vi "galvo_set_channels.vi"(8 "error in (no error)":errorcluster, 9 "y_channel":tag, 10 "x_channel":tag, 11 "galvo in":refnum<class "galvo.lvclass">) -> (0 "error out":errorcluster, 3 "galvo out":refnum<class "galvo.lvclass">)   [LabVIEW 2015, in "galvo.lvclass"]
uses:
  galvo.lvclass
  galvo.lvclass/galvo.ctl
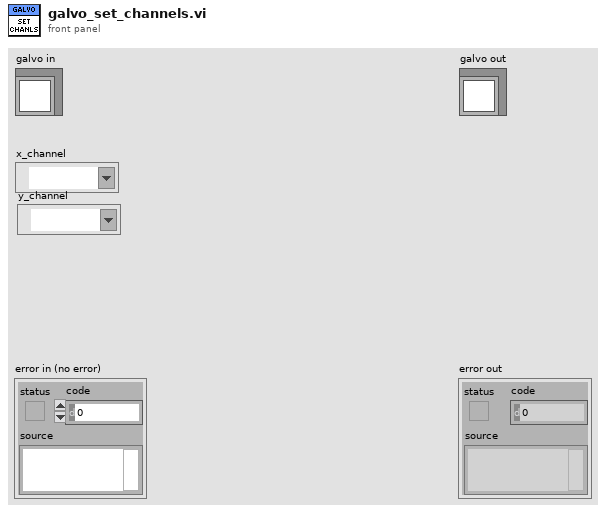
[diagram p1: front panel]
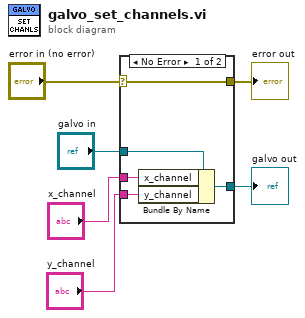
[diagram p0: block diagram]
diagram:
  n1 = case shown="No Error" "error in (no error)" {
    selector: "error in (no error)" -> [w11 w13]
    tunnel: [w11 w13] -> w5
    tunnel: [w7 w12] -> w3
    tunnel: "galvo in" -> [w8 w12]
    tunnel: "x_channel" -> [w10 _]
    tunnel: "y_channel" -> [w9 _]
    frame No Error {
      n2 = Bundle By Name(cluster=w8, "x_channel"=w10, "y_channel"=w9) -> (w7:refnum<class "galvo.lvclass">)
    }
    frame Error {
    }
  }
  "error out" <- w5
  "galvo out" <- w3
